vi "Flow Control.vi"(9 "input valid (nc)":bool=TRUE, 11 "rx core":refnum<class "niUSRP Rx Core v1 FPGA.lvclass">, 12 "ready for output (t)":bool=TRUE, 13 "trigger":bool) -> (10 "output valid":bool, 14 "ready for input (nc)":bool, 15 "rx core":refnum<class "niUSRP Rx Core v1 FPGA.lvclass">)   [LabVIEW 2025, in "niUSRP Rx Core v1 FPGA.lvclass"]
uses:
  niUSRP Rx Core v1 FPGA.lvclass
  niUSRP Rx Core v1 FPGA.lvclass/niUSRP Rx Core v1 FPGA.ctl
  <vilib>/rvi/DataTransferAndStorage/Container/Common/niFpgaContainerExecOnDevCompGetState.vi
  <vilib>/rvi/Emulation/niFpgaEmulationIsFPGAContextNoSignature.vi
  <vilib>/rvi/DataTransferAndStorage/Container/Common/niFpgaContainerGetUniqueNameForEmu.vi
  <vilib>/rvi/Memory/Memory_Emulation/niFpgaMemoryEmulationCacheClearOnFirstRun.vi
  <vilib>/rvi/Memory/Memory_Emulation/nirvimemoryEmulationManagerCache_MakeExclusive.vi
  <vilib>/rvi/Memory/Memory_Emulation/niFpgaMemoryEmulationValidateCache.vi
  <vilib>/rvi/Memory/Memory_Emulation/nirvimemoryEmulationManagerCache_InsertValue.vi
  <vilib>/Utility/error.llb/Clear Errors.vi
  <vilib>/rvi/Memory/Memory_Emulation/nirvimemoryEmulationManagerCache_ReleaseExclusive.vi
  <vilib>/rvi/Memory/Memory_Emulation/nirvimemoryEmulationManagerCache_GetValue.vi
  <vilib>/rvi/Memory/Memory_Emulation/nirvimemoryEmulationManagerCache_SetValue.vi
  <vilib>/rvi/Emulation/niFpgaProcessEmulError.vi
  <vilib>/rvi/Emulation/niFpgaSctlEmulationGetInTimedLoop.vi
  <vilib>/rvi/DataTransferAndStorage/Container/XNode/niFpgaContainer.xnode
  <vilib>/rvi/DataTransferAndStorage/Register/Emulation/niFpgaRegisterEmulationRefIn.vi
  <instrlib>/_niInstr/Basic Elements/v1/FPGA/niInstr Basic Elements v1 FPGA.lvlib
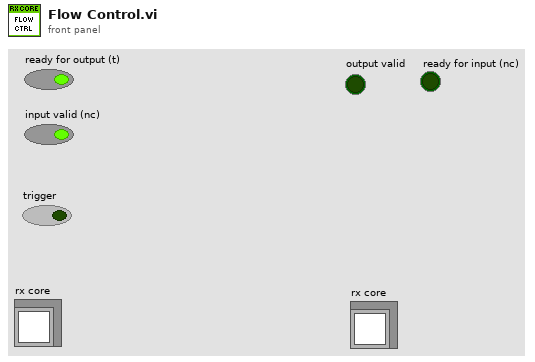
[diagram p1: front panel]
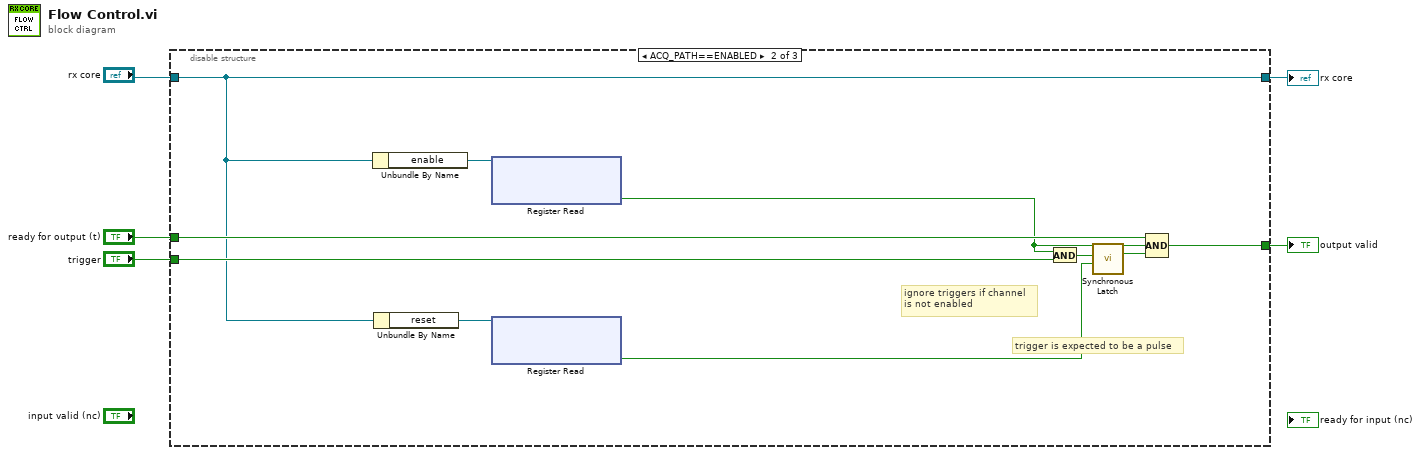
[diagram p0: block diagram]
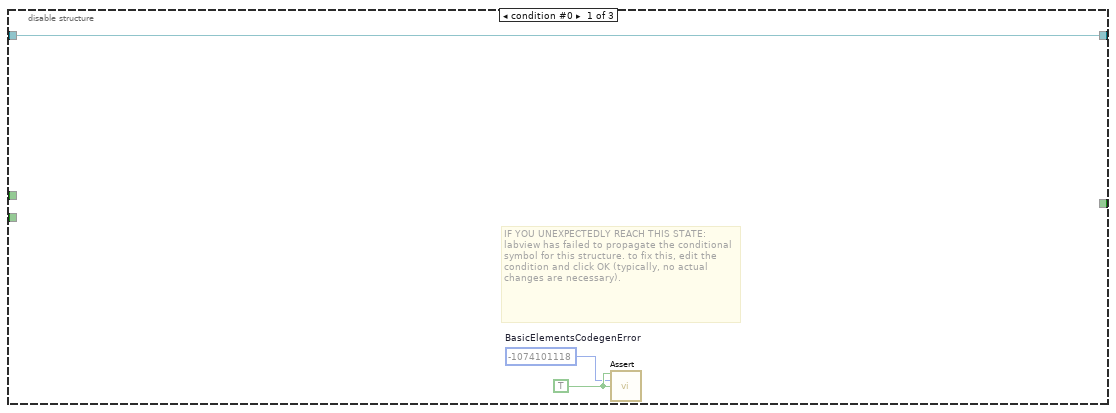
[diagram p2: hidden frame]
diagram:
  n1 = disable-structure shown="ACQ_PATH==ENABLED" {
    disable-tunnel: "rx core" -> [w6 w15 w19]
    disable-tunnel: [w6 w15 w19] -> w4
    disable-tunnel: [_ w16 _] -> w3
    disable-tunnel: "ready for output (t)" -> [_ w17 _]
    disable-tunnel: "trigger" -> [_ w18 _]
    frame condition #0 {
      w8 = TRUE ("assert")
      w7 = -1074101118  # BasicElementsCodegenError
      # "IF YOU UNEXPECTEDLY REACH THIS STATE:\nlabview has failed to propagate the conditional symbol for this structure. to fix this, edit the condition and click OK (typically, no actual changes are necessary)."
      n2 = call <instrlib>:"Assert.vi"("assert"=w8, "error code"=w7, "enable show error"=w8) -> ()  [unwired: 13 in]
    }
    frame condition #1 (active) {
      # "ignore triggers if channel\nis not enabled"
      # "trigger is expected to be a pulse"
      n3 = Unbundle By Name(w15) -> ("enable"=w14:refnum<k21>)
      n4 = Unbundle By Name(w15) -> ("reset"=w13:refnum<k21>)
      n5 = xnode ("Register Read")("Register In"=w14) -> ("Data"=w10:bool)  [unwired: 1 out]
      n6 = xnode ("Register Read")("Register In"=w13) -> ("Data"=w11:bool)  [unwired: 1 out]
      n7 = And(x=w10, y=w18) -> (x .and. y?=w12:bool)
      n8 = call <instrlib>:"Synchronous Latch.vi"("clear"=w11, "set"=w12) -> ("out"=w9:bool)  [unwired: 9 in]
      n9 = Compound Arithmetic op=AND(w17, w10, w9) -> (w16:bool)
    }
    frame condition #2 {
    }
  }
  "rx core" <- w4
  "output valid" <- w3
